vi "Self Configure.vi"(8 "error in":errorcluster, 11 "DIG_IO in":refnum<class "DIG_IO.lvclass">) -> (0 "error out":errorcluster, 3 "DIG_IO out":refnum<class "DIG_IO.lvclass">)   [LabVIEW 2019, in "DIG_IO.lvlib" / "DIG_IO.lvclass"]
uses:
  Library/DIG_IO.lvclass
  Custom Controls/Configuration Keys.ctl
  Library/DIG_IO.lvclass/DIG_IO.ctl
  builds/Instruments/Instruments.lvlibp/Library/Instruments.lvclass
  builds/Tools/Config.lvlibp/Config.lvclass
  C:/Users/Public/Documents/Development/builds/Tools/Config.lvlibp/Config.lvclass
panel:
  in  "Configuration Keys":T1
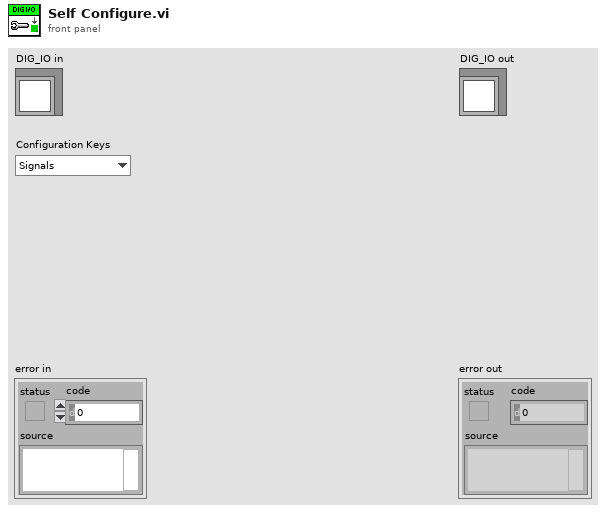
[diagram p1: front panel]
types:
  T1 = typedef "DIG_IO.lvlib/DIG_IO.lvclass/Configuration Keys.ctl" = enum16{"Signals", "CompactLogging"}
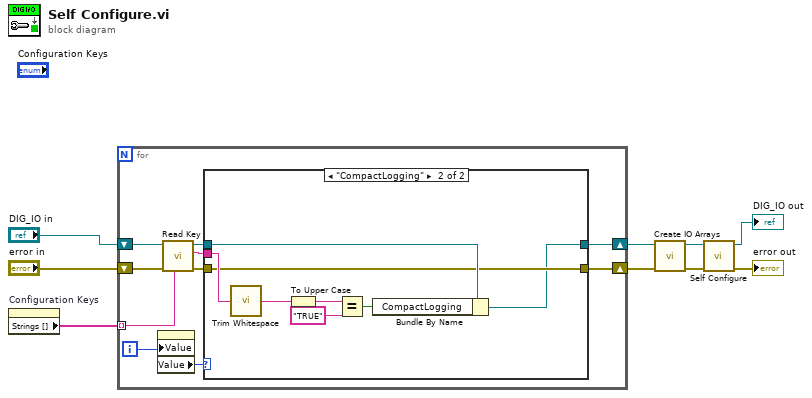
[diagram p0: block diagram]
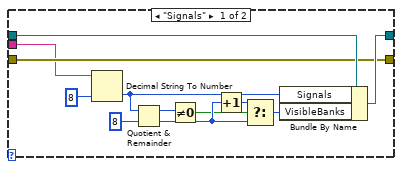
[diagram p2: hidden frame]
diagram:
  n1 = property on="Configuration Keys" class="Enum (strict)"() -> ("Strings []"=w5:string[])  [unwired: 2 in, 2 out]
  n2 = for {
    tunnel: w5 -> [w13] mode=indexing
    shift-right: [w16] -> w2
    shift-left: "DIG_IO in" -> [w14]
    shift-right: [w17] -> w1
    shift-left: "error in" -> [w15]
    i -> [w19]
    n3 = property on="Configuration Keys" class="Enum (strict)"("Value"=w19) -> ("Value"=w18:T1)  [unwired: 2 in, 2 out]
    n4 = call "Read Key.vi"("Key Name"=w13, "error in"=w15, "Config in"=w14) -> ("error out"=w11:errorcluster, "Key Value"=w10:string, "Config out"=w12:refnum<class "DIG_IO.lvclass">)  [unwired: 6 in]
    n5 = case shown="\"CompactLogging\"" w18 {
      tunnel: [w21 w34] -> w17
      tunnel: [w31 w33] -> w16
      tunnel: w12 -> [w22 w35]
      tunnel: w11 -> [w21 w34]
      tunnel: w10 -> [w20 w39]
      frame "Signals" {
        n6 = Decimal String To Number(string=w20, default (0L)=u8 8 ("y")) -> (number=w30:u8)  [unwired: 1 in, 1 out]
        n7 = Quotient & Remainder(x=w30, y=u8 8) -> (x-y*floor(x/y)=w25:u8, floor(x/y)=w27:u8)
        n8 = Not Equal To 0?(x=w25) -> (x != 0?=w24:bool)
        n9 = Increment(x=w27) -> (x+1=w28:u8)
        n10 = Select(t=w28, s=w24, f=w27) -> (s? t:f=w26:u8)
        n11 = Bundle By Name(cluster=w22, "Signals"=w30, "VisibleBanks"=w26) -> (w31:refnum<class "DIG_IO.lvclass">)
      }
      frame "CompactLogging" {
        n12 = call <vilib>:"Trim Whitespace.vi"("string"=w39) -> ("trimmed string"=w38:string)  [unwired: 1 in]
        n13 = To Upper Case(1:w38) -> (0:w37:string)
        n14 = Equal?(x=w37, y="TRUE") -> (x = y?=w32:bool)
        n15 = Bundle By Name(cluster=w35, "CompactLogging"=w32) -> (w33:refnum<class "DIG_IO.lvclass">)
      }
    }
  }
  n16 = call "Create IO Arrays.vi"("error in"=w1, "DIG_IO in"=w2) -> ("error out"=w8:errorcluster, "DIG_IO out"=w9:refnum<class "DIG_IO.lvclass">)  [unwired: 8 in]
  n17 = call-parent "Self Configure.vi"("error in"=w8, "Instruments in"=w9) -> ("error out"=→"error out":errorcluster, "Instruments out"=→"DIG_IO out":refnum<class "DIG_IO.lvclass">)  [unwired: 8 in]
